vi "Driver Pattern Exists.vi"(11 "File pattern":string="niscope*") -> (3 "file or folder exists?":bool)   [LabVIEW 2016]
uses:
  <vilib>/Utility/sysdir.llb/System Directory Type.ctl
panel:
  out "All Files in Dir":path[](array[path])
  out "system directory":path
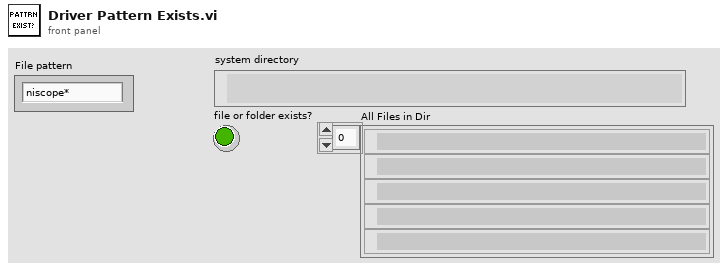
[diagram p1: front panel]
types:
  T1 = typedef "System Directory Type.ctl" = i32
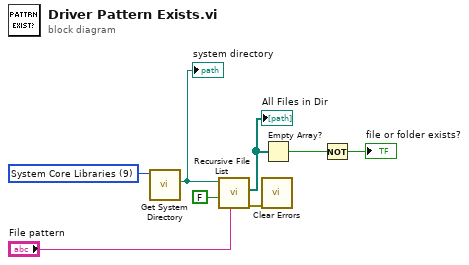
[diagram p0: block diagram]
diagram:
  w8 = T1 9 items=["User Home"=0, "User Desktop"=1, "User Documents"=2, "User Application Data"=3, "User Preferences"=4, "User Temporary"=5, "Public Documents"=6, "Public Application Data"=7, "Public Preferences"=8, "Public Cache"=13, "System Core Libraries"=9, "System Installed Libraries"=10, "Application Files"=11, "Boot Volume Root"=12] ("system directory type")
  n1 = call <vilib>:"Get System Directory.vi"("system directory type"=w8) -> ("system directory"=w7:path)  [unwired: 10 in]
  "system directory" <- w7
  n2 = call <vilib>:"Recursive File List.vi"("pattern"="File pattern", "Continue Recursing on Error? (F)"=FALSE, "Folder Path"=w7) -> ("error out"=w5:errorcluster, "All Files in Dir"=w4:path[])  [unwired: 4 in, 3 out]
  "All Files in Dir" <- w4
  n3 = call <vilib>:"Clear Errors.vi"("error in (no error)"=w5) -> ()  [unwired: 5 in, 2 out]
  n4 = Empty Array?(array=w4) -> (empty?=w3:bool)
  n5 = Not(x=w3) -> (.not. x?=→"file or folder exists?":bool)
